vi "prueba_digital.vi"() -> ()   [LabVIEW 2025]
panel:
  in  "Pin":u8=4 min=4 max=40
  in  "error in (no error)":errorcluster
  out "error out":errorcluster
  out "Valor":bool
  in  "Pin W":u8=4 min=4 max=40
  in  "stop":bool
  in  "VISA resource name":refnum<visa-resource-name>
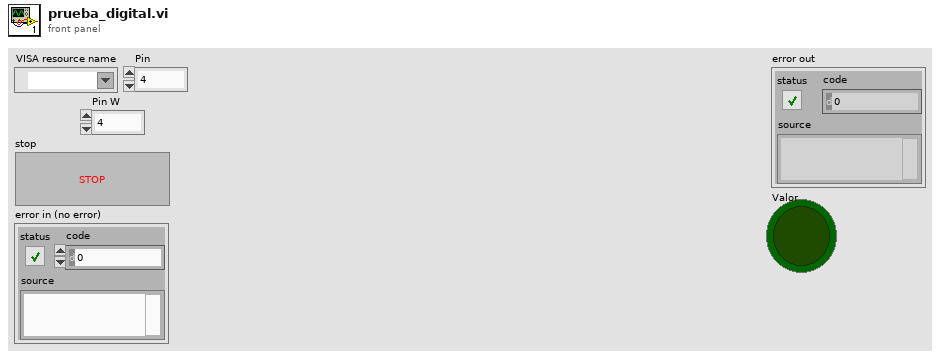
[diagram p1: front panel]
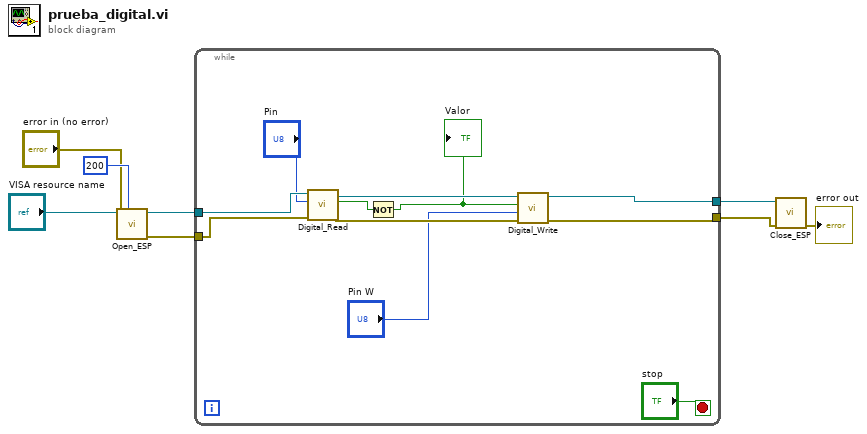
[diagram p0: block diagram]
diagram:
  n1 = call "Open_ESP.vi"("timeout (10sec)"=u32 200, "error in (no error)"="error in (no error)", "VISA resource name"="VISA resource name") -> ("error out"=w6:errorcluster, "VISA resource name out"=w7:refnum<visa-resource-name>)  [unwired: 7 in]
  n2 = while {
    tunnel: w7 -> [w19]
    tunnel: w6 -> [w12]
    tunnel: [w17] -> w4
    tunnel: [w16] -> w3
    stop <- "stop" stop-if-true
    n3 = call "Digital_Read.vi"("error in (no error)"=w12, "Pin"="Pin", "VISA resource name"=w19) -> ("error out"=w15:errorcluster, "Valor"=w10:bool, "VISA resource name out"=w14:refnum<visa-resource-name>)  [unwired: 6 in]
    n4 = Not(x=w10) -> (.not. x?=w9:bool)
    "Valor" <- w9
    n5 = call "Digital_Write.vi"("error in (no error)"=w15, "Pin"="Pin W", "Estado"=w9, "VISA resource name"=w14) -> ("error out"=w16:errorcluster, "VISA resource name out"=w17:refnum<visa-resource-name>)  [unwired: 6 in]
  }
  n6 = call "Close_ESP.vi"("error in (no error)"=w3, "VISA resource name"=w4) -> ("error out"=→"error out":errorcluster)  [unwired: 9 in]
